vi "Phasor Update (g,s) on UC to New Frequency.vi"(8 "Error In":errorcluster, 9 "New Phasor Frequency":dbl[unit], 10 "Lifetime":dbl[unit], 11 "Phasor in":T1) -> (0 "Error Out":errorcluster, 3 "Phasor out":T1)   [LabVIEW 2021, in "Phasor.lvlib"]
uses:
  Phasor.lvlib
  Phasor (g, s).ctl
  <vilib>/ErrorRing/Error Ring.xnode
  <vilib>/Utility/error.llb/Error Cluster From Error Code.vi
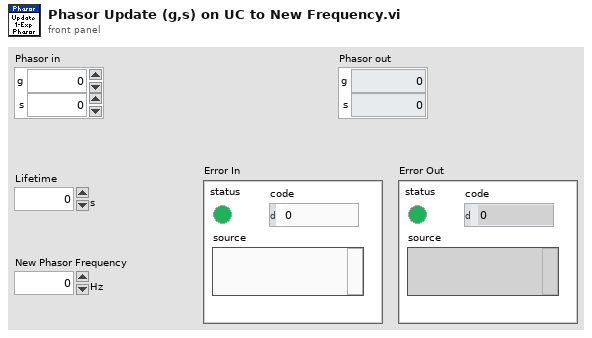
[diagram p1: front panel]
types:
  T1 = typedef "Phasor.lvlib/Phasor (g, s).ctl" = cluster{"g":dbl, "s":dbl}
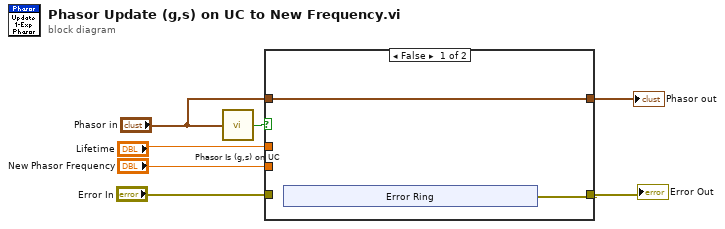
[diagram p0: block diagram]
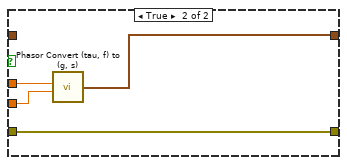
[diagram p2: hidden frame]
diagram:
  n1 = call "Phasor Is (g,s) on UC.vi"("Phasor (g, s)"="Phasor in") -> ("Is on UC?"=w7:bool)  [unwired: 8 in]
  n2 = case shown="False" w7 {
    tunnel: "Phasor in" -> [w9 _]
    tunnel: [w9 w15] -> w6
    tunnel: "Lifetime" -> [_ w17]
    tunnel: "New Phasor Frequency" -> [_ w16]
    tunnel: "Error In" -> [_ w14]
    tunnel: [w8 w14] -> w1
    frame False {
      n3 = xnode "Error Ring"() -> ("error out"=w8:errorcluster)
    }
    frame True {
      n4 = call "Phasor Convert (tau, f) to (g, s).vi"("Lifetime"=w17, "Phasor Frequency"=w16) -> ("Phasor (g, s)"=w15:T1)  [unwired: 5 in]
    }
  }
  "Phasor out" <- w6
  "Error Out" <- w1
